vi "Module Init.vi"(8 "error in (no error)":errorcluster, 11 "Status Submodule in":refnum<class "Status Submodule.lvclass">) -> (0 "error out":errorcluster, 3 "Status Submodule out":refnum<class "Status Submodule.lvclass">)   [LabVIEW 2020, in "VolatusSeq.lvlib" / "Status Submodule.lvclass"]
uses:
  Status Submodule.lvclass
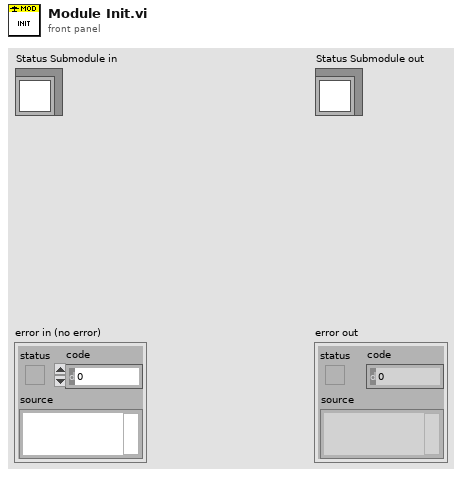
[diagram p1: front panel]
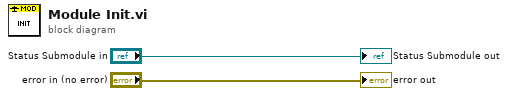
[diagram p0: block diagram]
diagram:
  "error out" <- "error in (no error)"
  "Status Submodule out" <- "Status Submodule in"
